vi "makevideofrompics.vi"() -> ()   [LabVIEW 2009]
panel:
  out "Total":i32
  in  "Frames Per Second":u32=2
  out "Image":T1(plugin-control)
  out "Color Palette out":cluster{"Red":u8, "Green":u8, "Blue":u8}[](array[cluster])
  out "String":string
  in  "File Options":T2 {"Optional Max Value" format="%.2f"; "Optional Min Value" format="%.2f"; "File Data Type" items=["1 bit", "2 bits", "4 bits", "8 bits", "16 bits (unsigned)", "16 bits (signed)", "16 bits (RGB chunky)", "24 bits (RGB chunky)", "24 bits (RGB planar)", "32 bits (unsigned)", "32 bits (signed)", "32 bits (RGB chunky)", "32 bits (float)", "48 bits (Complex 2x24 int)", "64 bits (Complex 2x32 float)", "32 bits (HSL)"]; "Read Raw File" items=["Don't Read Raw File ", "Read Raw File"]}
  out "Numeric":i32
  in  "index":i32
  out "Filter Names":string[](array[string])
  in  "AVI Path":path
  in  "Path":path
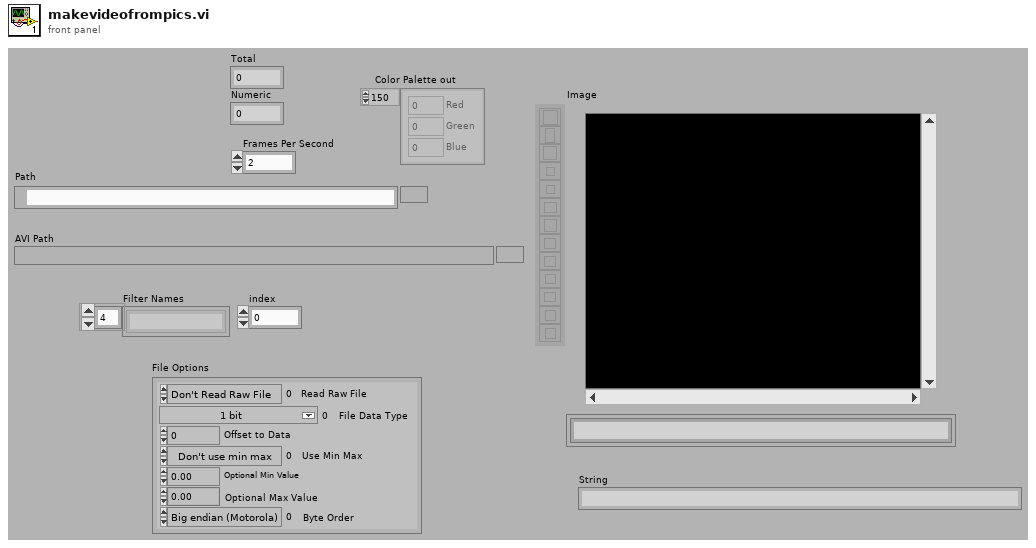
[diagram p1: front panel]
types:
  T1 = typedef "IMAQ Image.ctl" = refnum<image>
  T2 = cluster{"Read Raw File":i32, "File Data Type":u32, "Offset to Data":i32, "Use Min Max":enum32{"Don't use min max", "Use file values", "Use optional values"}, "Optional Min Value":sgl, "Optional Max Value":sgl, "Byte Order":enum32{"Big endian (Motorola)", "Little endian (Intel)"}}
  T3 = typedef "Image Type" = u32
  T4 = typedef "AviRefnum.ctl" = refnum<k1>
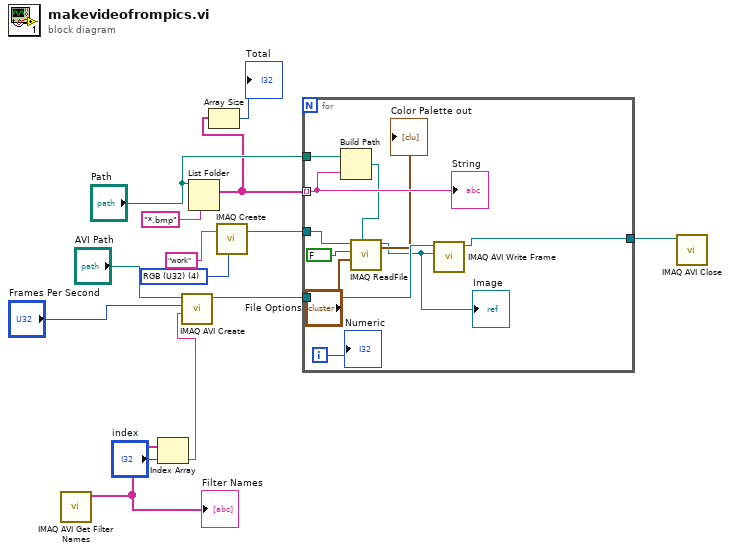
[diagram p0: block diagram]
diagram:
  w3 = T3 4 items=["Grayscale (U8)", "Grayscale (I16)", "Grayscale (SGL)", "Complex (CSG)", "RGB (U32)", "HSL (U32)", "RGB (U64)", "Grayscale (U16)"] ("Image Type")
  n1 = call "IMAQ AVI Get Filter Names"() -> ("Filter Names"=w14:string[])  [unwired: 10 in, 1 out]
  "Filter Names" <- w14
  n2 = Index Array(array=w14, index="index") -> (element=w6:string)
  n3 = call "IMAQ AVI Create"("Compression Filter"=w6, "Frames Per Second"="Frames Per Second", "AVI Path"="AVI Path") -> ("Avi Refnum"=w10:T4)  [unwired: 7 in, 1 out]
  n4 = List Folder(path="Path", pattern="*.bmp") -> (filenames=w2:string[])  [unwired: 2 in, 3 out]
  n5 = Array Size(array=w2) -> (size(s)=→"Total":i32)
  n6 = call "IMAQ Create"("Image Name"="work", "Image Type"=w3) -> ("New Image"=w11:T1)  [unwired: 3 in, 1 out]
  n7 = for {
    tunnel: w2 -> [w20] mode=indexing
    tunnel: w11 -> [w25]
    tunnel: w10 -> [w23]
    tunnel: [w22] -> w9
    tunnel: "Path" -> [w21]
    i -> [w18]
    n8 = Build Path(base path=w21, name or relative path=w20) -> (appended path=w19:path)
    n9 = call "IMAQ ReadFile"("File Path"=w19, "File Options"="File Options", "Load Color Palette? (No)"=FALSE, "Image"=w25) -> ("Image Out"=w15:T1, "Color Palette out"=→"Color Palette out":cluster{"Red":u8, "Green":u8, "Blue":u8}[])  [unwired: 3 in, 3 out]
    "Image" <- w15
    n10 = call "IMAQ AVI Write Frame"("Image"=w15, "Avi Refnum"=w23) -> ("Avi Refnum (duplicate)"=w22:T4)  [unwired: 8 in, 1 out]
    "Numeric" <- w18
    "String" <- w20
  }
  n11 = call "IMAQ AVI Close"("Avi Refnum"=w9) -> ()  [unwired: 10 in, 1 out]
